vi "Init Project Watcher.vi"(8 "error in (no error)":errorcluster, 11 "GVIWebProcessorApp in":refnum<class "GVIWebProcessorApp.lvclass">) -> (0 "error out":errorcluster, 3 "GVIWebProcessorApp out":refnum<class "GVIWebProcessorApp.lvclass">)   [LabVIEW 2020, in "PicoG-Processor.lvlib" / "GVIWebProcessorApp.lvclass"]
uses:
  GVIWebProcessorApp.lvclass
  GVIWebProcessorApp.lvclass/GVIWebProcessorApp.ctl
  Builds Updated Callback.vi
  WebProjectWatcher/WebProjectWatcher.lvclass
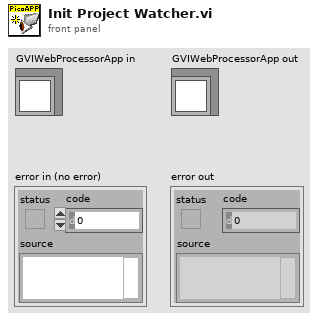
[diagram p1: front panel]
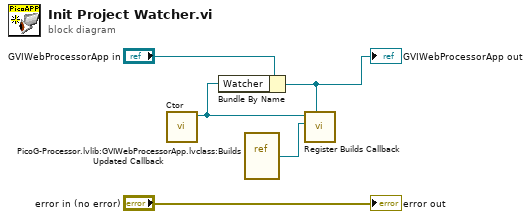
[diagram p0: block diagram]
diagram:
  n1 = call "Ctor.vi"() -> ("WebProjectWatcher out"=w3:refnum<class "WebProjectWatcher.lvclass">)  [unwired: 10 in, 1 out]
  n2 = Bundle By Name(cluster="GVIWebProcessorApp in", "Watcher"=w3) -> (w2:refnum<class "GVIWebProcessorApp.lvclass">)
  "GVIWebProcessorApp out" <- w2
  n3 = vi-ref "PicoG-Processor.lvlib:GVIWebProcessorApp.lvclass:Builds Updated Callback.vi"() -> (w1:refnum<vi>)
  n4 = call "Register Builds Callback.vi"("Owner"=w2, "Callback"=w1, "WebProjectWatcher in"=w3) -> ()  [unwired: 7 in, 2 out]
  "error out" <- "error in (no error)"
